vi "SEA_9811_RT_Driver_Tester.vi"() -> ()   [LabVIEW 2012]
uses:
  Typdefs/SEA9811_RT_conf_cluster.ctl
  <vilib>/userdefined/High Color/nirio_resource_hc.ctl
  FPGA/SEA-9811_ReceiverAndTransmitter/SubVIs/SEA-9811_ReceiverAndTransmitter_RCR.ctl
  FPGA/SEA-9811_ReceiverAndTransmitter/SubVIs/SEA-9811_ReceiverAndTransmitter_TCR.ctl
  FPGA/SEA-9811_ReceiverAndTransmitter/SubVIs/SEA-9811_ReceiverAndTransmitter_RSR.ctl
  Typdefs/ARINC word cluster.ctl
  Typdefs/ARINC word.ctl
  Typdefs/channel.ctl
  Typdefs/received word.ctl
  <vilib>/Platform/TimedLoop/XDataNode/timing_clust.ctl
  <vilib>/Platform/TimedLoop/XDataNode/nitl_modes.ctl
  <vilib>/Platform/TimedLoop/XDataNode/wakeup.ctl
  <vilib>/Platform/TimedLoop/XDataNode/XDataNode.xnode
  <vilib>/Platform/TimedLoop/XDataNode/XDNodeRunTimeDep.lvlib
panel:
  in  "Run FPGA?":bool
  in  "Period (ms)":i64=5
  out "Channels":T1[](array[typedef]) {"Received Words"."word" format="%.0o"; "Received Words"."timestamp" format="%#.10g"}
  in  "ARINC word in":T3 {"ARINC word" format="%032b"}
  out "error out":errorcluster
  in  "stop 2":bool
  out "Receiver Status Register (RSR)":T5={"RSR0: FIFO channel 0 empty"=TRUE, "RSR1: FIFO channel 1 empty"=TRUE, "RSR2: FIFO channel 2 empty"=TRUE, "RSR3: FIFO channel 3 empty"=TRUE, "RSR4: FIFO channel 4 empty"=TRUE, "RSR5: FIFO channel 5 empty"=TRUE, "RSR6: FIFO channel 6 empty"=TRUE, "RSR7: FIFO channel 7 empty"=TRUE, "RSR8: FIFO channel 0 full"=FALSE, "RSR9: FIFO channel 1 full"=FALSE, "RSR10: FIFO channel 2 full"=FALSE, "RSR11: FIFO channel 3 full"=FALSE, "RSR12: FIFO channel 4 full"=FALSE, "RSR13: FIFO channel 5 full"=FALSE, "RSR14: FIFO channel 6 full"=FALSE, "RSR15: FIFO channel 7 full"=FALSE}
  out "DMA Overflow":bool
  in  "stop":bool
  in  "SEA9811_conf_cluster":T6={"FPGA resource name"="RIO0", "Rx ch conf (0..7)"=[{"Rx Channel Number (0..7)"=0, "Rx Label Filter"={"Label 00"=0, "Label 01"=0, "Label 02"=0, "Label 03"=0, "Label 04"=0, "Label 05"=0, "Label 06"=0, "Label 07"=0, "Label 08"=0, "Label 09"=0, "Label 10"=0, "Label 11"=0, "Label 12"=0, "Label 13"=0, "Label 14"=0, "Label 15"=0}, "Receiver Control Register (RCR)"={"RCR0: Data rate = ARINC 429 High-Speed (0) or Low-Speed (1)"=FALSE, "RCR1: not used"=FALSE, "RCR2: Label recognition for this channel enabled (1) or disabled (0)"=FALSE, "RCR3: Receiver channel disabled (1) or enabled (0)"=FALSE, "RCR4: Odd parity check for this channel enabled (1) or disabled (0"=FALSE, "RCR5: Receiver normal operation (1) or loopback mode (0)"=TRUE, "RCR6: Receiver Decoder disabled (0) or enabled (1) \n-> ARINC bits 10 and 9 must match RCR7 and RCR8"=FALSE, "RCR7: If receiver decoder is enabled (RCR6=1), \nthe ARINC bit 10 must match this bit"=FALSE, "RCR8: If receiver decoder is enabled (RCR6=1), \nthe ARINC bit 9 must match this bit"=FALSE, "RCR9: Label bit order for this channel non-reversed (1) \nor reversed (0)"=FALSE, "RCR10: not used"=FALSE, "RCR11: not used"=FALSE, "RCR12: not used"=FALSE, "RCR13: not used"=FALSE, "RCR14: not used"=FALSE, "RCR15: not used"=FALSE}}, {"Rx Channel Number (0..7)"=3, "Rx Label Filter"={"Label 00"=23, "Label 01"=34, "Label 02"=0, "Label 03"=0, "Label 04"=0, "Label 05"=0, "Label 06"=0, "Label 07"=0, "Label 08"=0, "Label 09"=0, "Label 10"=0, "Label 11"=0, "Label 12"=0, "Label 13"=0, "Label 14"=0, "Label 15"=0}, "Receiver Control Register (RCR)"={"RCR0: Data rate = ARINC 429 High-Speed (0) or Low-Speed (1)"=FALSE, "RCR1: not used"=FALSE, "RCR2: Label recognition for this channel enabled (1) or disabled (0)"=FALSE, "RCR3: Receiver channel disabled (1) or enabled (0)"=FALSE, "RCR4: Odd parity check for this channel enabled (1) or disabled (0"=FALSE, "RCR5: Receiver normal operation (1) or loopback mode (0)"=TRUE, "RCR6: Receiver Decoder disabled (0) or enabled (1) \n-> ARINC bits 10 and 9 must match RCR7 and RCR8"=FALSE, "RCR7: If receiver decoder is enabled (RCR6=1), \nthe ARINC bit 10 must match this bit"=FALSE, "RCR8: If receiver decoder is enabled (RCR6=1), \nthe ARINC bit 9 must match this bit"=FALSE, "RCR9: Label bit order for this channel non-reversed (1) \nor reversed (0)"=FALSE, "RCR10: not used"=FALSE, "RCR11: not used"=FALSE, "RCR12: not used"=FALSE, "RCR13: not used"=FALSE, "RCR14: not used"=FALSE, "RCR15: not used"=FALSE}}, {"Rx Channel Number (0..7)"=5, "Rx Label Filter"={"Label 00"=2, "Label 01"=3, "Label 02"=0, "Label 03"=0, "Label 04"=0, "Label 05"=0, "Label 06"=0, "Label 07"=0, "Label 08"=0, "Label 09"=0, "Label 10"=0, "Label 11"=0, "Label 12"=0, "Label 13"=0, "Label 14"=0, "Label 15"=0}, "Receiver Control Register (RCR)"={"RCR0: Data rate = ARINC 429 High-Speed (0) or Low-Speed (1)"=FALSE, "RCR1: not used"=FALSE, "RCR2: Label recognition for this channel enabled (1) or disabled (0)"=FALSE, "RCR3: Receiver channel disabled (1) or enabled (0)"=FALSE, "RCR4: Odd parity check for this channel enabled (1) or disabled (0"=FALSE, "RCR5: Receiver normal operation (1) or loopback mode (0)"=TRUE, "RCR6: Receiver Decoder disabled (0) or enabled (1) \n-> ARINC bits 10 and 9 must match RCR7 and RCR8"=FALSE, "RCR7: If receiver decoder is enabled (RCR6=1), \nthe ARINC bit 10 must match this bit"=FALSE, "RCR8: If receiver decoder is enabled (RCR6=1), \nthe ARINC bit 9 must match this bit"=FALSE, "RCR9: Label bit order for this channel non-reversed (1) \nor reversed (0)"=FALSE, "RCR10: not used"=FALSE, "RCR11: not used"=FALSE, "RCR12: not used"=FALSE, "RCR13: not used"=FALSE, "RCR14: not used"=FALSE, "RCR15: not used"=FALSE}}], "Transmitter Control Register (TCR)"={"TCR0: not used"=FALSE, "TCR1: not used"=FALSE, "TCR2: not used"=FALSE, "TCR3: Transmitter Parity Bit Enable: 32nd bit is parity (1) or data (0)"=FALSE, "TCR4: not used"=FALSE, "TCR5: not used"=FALSE, "TCR6: not used"=FALSE, "TCR7: not used"=FALSE, "TCR8: not used"=FALSE, "TCR9: Transmitter Parity Select: odd parity (0) or even parity (1)"=FALSE, "TCR10: Transmitter Data Rate: ARINC 429 high-speed (0) or low-speed (1)"=FALSE, "TCR11: ARINC Label Bit Order: label bit order reversed (0) or not reversed (1)"=FALSE, "TCR12: Disable Line Driver: normal operation (0) or transmitter disabled (1)"=FALSE, "TCR13: Tansmit whenever data is available in FIFO (1) or only start by instruction \"Enable Transmission\" (0)"=TRUE, "TCR14: not used"=FALSE, "TCR15: not used"=FALSE}, "Bitfile Path"=path "c:/SEA-9811_ReceiverAndTransmitter_FPGA_IO_simulated.vi.lvbitx"}
  # "Run FPGA VI directly for interactive execution! Otherwise set Run FPGA? to TRUE"
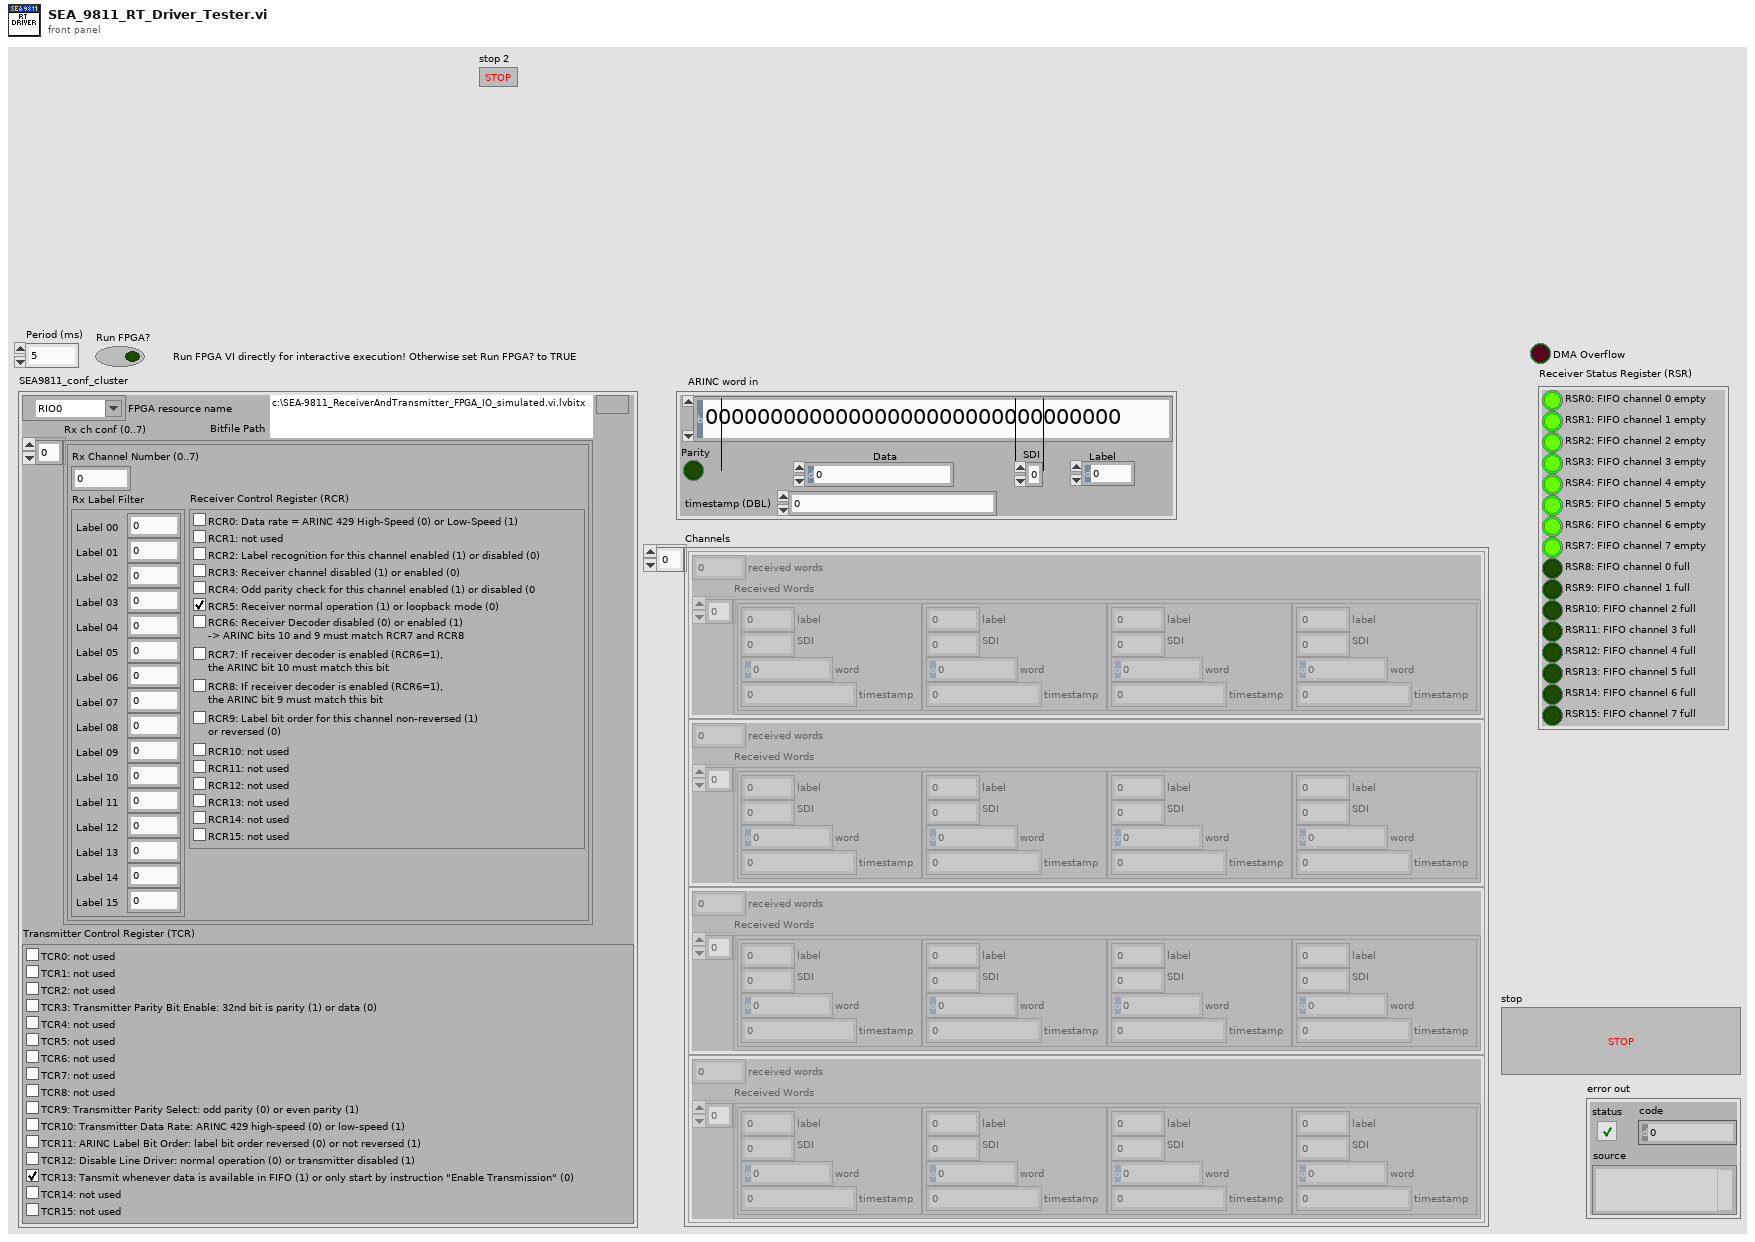
[diagram p1: front panel]
types:
  T1 = typedef "channel.ctl" = cluster{"received words":u32, "Received Words":T2[]}
  T2 = typedef "received word.ctl" = cluster{"label":u8, "SDI":u8, "word":u32, "timestamp":dbl}
  T3 = typedef "ARINC word cluster.ctl" = cluster{"ARINC word":T4, "Label":u8, "SDI":u8, "Data":u32, "Parity":bool, "timestamp (DBL)":dbl}
  T4 = typedef "ARINC word.ctl" = u32
  T5 = typedef "SEA-9811_ReceiverAndTransmitter_RSR.ctl" = cluster{"RSR0: FIFO channel 0 empty":bool, "RSR1: FIFO channel 1 empty":bool, "RSR2: FIFO channel 2 empty":bool, "RSR3: FIFO channel 3 empty":bool, "RSR4: FIFO channel 4 empty":bool, "RSR5: FIFO channel 5 empty":bool, "RSR6: FIFO channel 6 empty":bool, "RSR7: FIFO channel 7 empty":bool, "RSR8: FIFO channel 0 full":bool, "RSR9: FIFO channel 1 full":bool, "RSR10: FIFO channel 2 full":bool, "RSR11: FIFO channel 3 full":bool, "RSR12: FIFO channel 4 full":bool, "RSR13: FIFO channel 5 full":bool, "RSR14: FIFO channel 6 full":bool, "RSR15: FIFO channel 7 full":bool}
  T6 = typedef "SEA9811_RT_conf_cluster.ctl" = cluster{"FPGA resource name":T7, "Rx ch conf (0..7)":cluster{"Rx Channel Number (0..7)":u8, "Rx Label Filter":cluster{"Label 00":u8, "Label 01":u8, "Label 02":u8, "Label 03":u8, "Label 04":u8, "Label 05":u8, "Label 06":u8, "Label 07":u8, "Label 08":u8, "Label 09":u8, "Label 10":u8, "Label 11":u8, "Label 12":u8, "Label 13":u8, "Label 14":u8, "Label 15":u8}, "Receiver Control Register (RCR)":T8}[], "Transmitter Control Register (TCR)":T9, "Bitfile Path":path}
  T7 = typedef "nirio_resource_hc.ctl" = tag
  T8 = typedef "SEA-9811_ReceiverAndTransmitter_RCR.ctl" = cluster{"RCR0: Data rate = ARINC 429 High-Speed (0) or Low-Speed (1)":bool, "RCR1: not used":bool, "RCR2: Label recognition for this channel enabled (1) or disabled (0)":bool, "RCR3: Receiver channel disabled (1) or enabled (0)":bool, "RCR4: Odd parity check for this channel enabled (1) or disabled (0":bool, "RCR5: Receiver normal operation (1) or loopback mode (0)":bool, "RCR6: Receiver Decoder disabled (0) or enabled (1) \n-> ARINC bits 10 and 9 must match RCR7 and RCR8":bool, "RCR7: If receiver decoder is enabled (RCR6=1), \nthe ARINC bit 10 must match this bit":bool, "RCR8: If receiver decoder is enabled (RCR6=1), \nthe ARINC bit 9 must match this bit":bool, "RCR9: Label bit order for this channel non-reversed (1) \nor reversed (0)":bool, "RCR10: not used":bool, "RCR11: not used":bool, "RCR12: not used":bool, "RCR13: not used":bool, "RCR14: not used":bool, "RCR15: not used":bool}
  T9 = typedef "SEA-9811_ReceiverAndTransmitter_TCR.ctl" = cluster{"TCR0: not used":bool, "TCR1: not used":bool, "TCR2: not used":bool, "TCR3: Transmitter Parity Bit Enable: 32nd bit is parity (1) or data (0)":bool, "TCR4: not used":bool, "TCR5: not used":bool, "TCR6: not used":bool, "TCR7: not used":bool, "TCR8: not used":bool, "TCR9: Transmitter Parity Select: odd parity (0) or even parity (1)":bool, "TCR10: Transmitter Data Rate: ARINC 429 high-speed (0) or low-speed (1)":bool, "TCR11: ARINC Label Bit Order: label bit order reversed (0) or not reversed (1)":bool, "TCR12: Disable Line Driver: normal operation (0) or transmitter disabled (1)":bool, "TCR13: Tansmit whenever data is available in FIFO (1) or only start by instruction \"Enable Transmission\" (0)":bool, "TCR14: not used":bool, "TCR15: not used":bool}
  T10 = typedef "SEA9811_RT_data_cluster.ctl" = cluster{"FPGA VI Reference":T11, "Channels":T1[], "FPGA FP":T12, "Tx":cluster{"Tx Refs (Data,Trig)":T13[], "Values":dbl[]}}
  T11 = typedef "FPGA ref.ctl" = refnum<k20>
  T12 = typedef "SEA9811_FPGA_FP_Addresses.ctl" = cluster{"FPGA Interface Base on":refnum<class "FPGA Interface Base.lvclass">, "FPGA Session":u32, "RT time (ns)":u32, "DMA Overflow":u32, "Elements in FIFO":u32, "Rx Status":u32, "Rx Data (FIFO)":u32, "Tx Data":u32, "Transmit Data":u32}
  T13 = typedef "Custom Device API.lvlib/Block Data Reference.ctl" = cluster{"Data Reference":T14, "Offset":i32, "Length":i32}
  T14 = typedef "Custom Device API.lvlib/Data Reference.ctl" = i32
  T15 = typedef "XDNodeRunTimeDep.lvlib/timing_clust.ctl" = cluster{"Expected End [f-1]":u64, "Actual End [f-1]":u64, "Finished Late? [f-1]":bool, "Expected End [i-1]":u64, "Actual End [i-1]":u64, "Finished Late? [i-1]":bool, "Expected Start [i]":u64, "Actual Start [i]":u64, "Expected Start [f]":u64, "Actual Start [f]":u64, "Source Name":string, "Structure Name":string, "Period":i64, "Deadline":i64, "Offset":i64, "Start":i64, "Priority":i32, "Timeout":i32, "Mode":T16, "Wakeup Reason":T17, "Error":errorcluster, "Source Type":string, "Secondary Source Type":string, "Global End Time":u64, "Global Start Time":u64, "Frame Duration":u64, "Iteration Duration":u64, "Assigned CPU":i32, "I/O Scan Engine Mode":u32}
  T16 = typedef "XDNodeRunTimeDep.lvlib/nitl_modes.ctl" = enum32{"No Change", "Process missed periods, maintain original phase", "Discard missed periods, maintain original phase", "Process missed periods, ignore original phase", "Discard missed periods, ignore original phase"}
  T17 = typedef "XDNodeRunTimeDep.lvlib/wakeup.ctl" = enum32{"Normal", "Aborted", "Asynchronous wakeup", "Timing source error", "Timed loop error", "Timeout"}
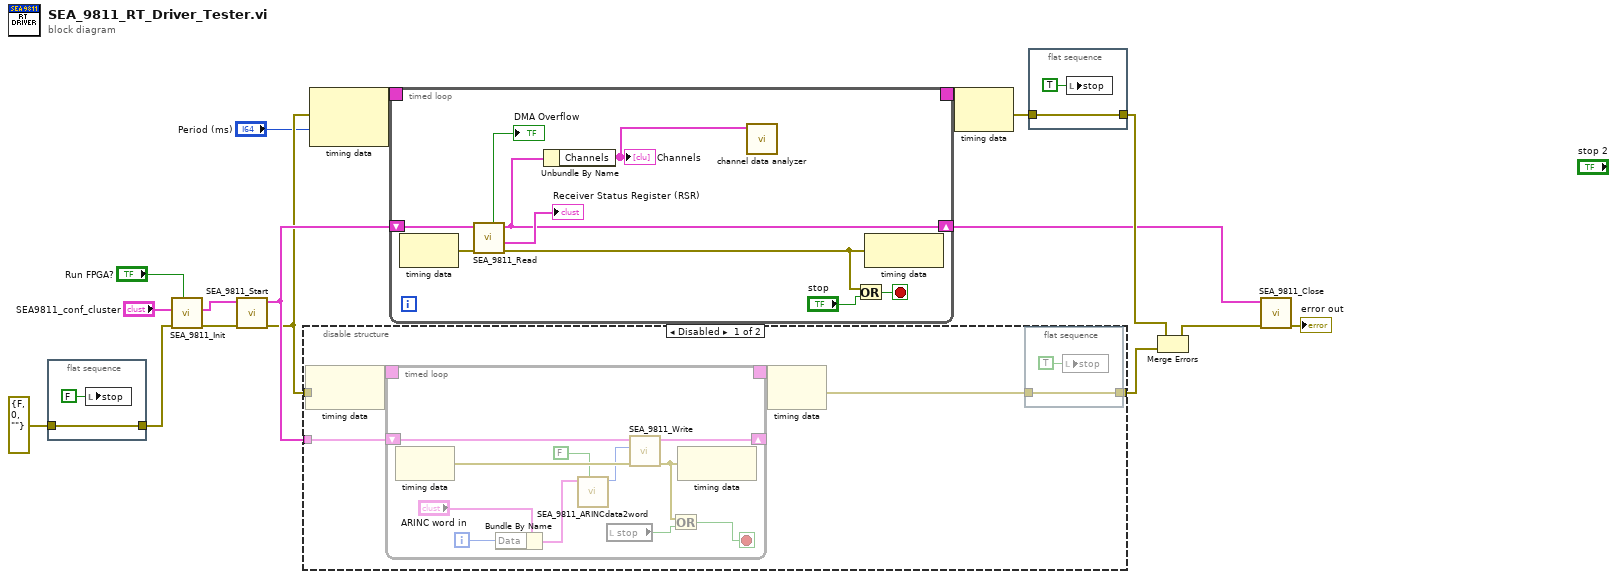
[diagram p0: block diagram]
diagram:
  n1 = flat-sequence {
    tunnel: errorcluster {"status"=FALSE, "code"=0, "source"=""} ("error in") -> [w18]
    tunnel: [w18] -> w11
    frame #0 {
      n2 = local write "stop"(FALSE ("stop")) -> ()
    }
  }
  n3 = call "SEA_9811_Init.vi"("Run?"="Run FPGA?", "error in"=w11, "SEA9811_conf_cluster"="SEA9811_conf_cluster") -> ("error out"=w17:errorcluster, "SEA9811_RT_data out"=w3:T10)  [unwired: 6 in, 1 out]
  n4 = call "SEA_9811_Start.vi"("error in (no error)"=w17, "SEA9811_RT_data in"=w3) -> ("error out"=w13:errorcluster, "SEA9811_RT_data out"=w16:T10)  [unwired: 8 in]
  n5 = disable-structure shown="Disabled" {
    disable-tunnel: w16 -> [w23 _]
    disable-tunnel: w13 -> [w22 w49]
    disable-tunnel: [w20 w49] -> w8
    frame Disabled {
      n6 = node-c288(w22) -> (w25:T15)
      n7 = timed-loop {
        timing: w25 -> [_]
        timing-out: [_] -> w24
        shift-right: [w31] -> _
        shift-left: w23 -> [w36]
        i -> [w29]
        stop <- w32 stop-if-true
        n8 = node-c288() -> (w35:errorcluster)  [unwired: 1 in]
        n9 = Bundle By Name(cluster="ARINC word in", "Data"=w29) -> (w27:T3)
        n10 = call "SEA_9811_ARINCdata2word.vi"("Reverse label bits"=FALSE, "ARINC word in"=w27) -> ("ARINC word out"=w30:T4)  [unwired: 8 in, 1 out]
        n11 = local read "stop"() -> (w34:bool)
        n12 = call "SEA_9811_Write.vi"("error in (no error)"=w35, "Tx Data"=w30, "SEA9811_RT_data in"=w36) -> ("error out"=w33:errorcluster, "SEA9811_RT_data out"=w31:T10)  [unwired: 7 in]
        n13 = Or(x=w33, y=w34) -> (x .or. y?=w32:bool)
        n14 = node-c288(w33) -> ()  [unwired: 1 out]
      }
      n15 = node-c288(w24) -> (w21:errorcluster)
      n16 = flat-sequence {
        tunnel: w21 -> [w47]
        tunnel: [w47] -> w20
        frame #0 {
          n17 = local write "stop"(TRUE ("stop")) -> ()
        }
      }
    }
    frame Enabled {
      # "write not implemented in dynamic bitfile version"
    }
  }
  n18 = node-c288(w13, "Period (ms)") -> (w15:T15)
  n19 = timed-loop {
    timing: w15 -> [_]
    timing-out: [_] -> w14
    shift-right: [w51] -> w6
    shift-left: w16 -> [w58]
    stop <- w55 stop-if-true
    n20 = node-c288() -> (w57:errorcluster)  [unwired: 1 in]
    n21 = call "SEA_9811_Read.vi"("error in (no error)"=w57, "SEA9811_RT_data in"=w58) -> ("error out"=w52:errorcluster, "Receiver Status Register (RSR)"=→"Receiver Status Register (RSR)":T5, "SEA9811_RT_data out"=w51:T10, "DMA Overflow"=→"DMA Overflow":bool)  [unwired: 6 in]
    n22 = Unbundle By Name(w51) -> ("Channels"=w50:T1[])
    "Channels" <- w50
    n23 = call "channel data analyzer.vi"("Channels"=w50) -> ()  [unwired: 11 in]
    n24 = Or(x=w52, y="stop") -> (x .or. y?=w55:bool)
    n25 = node-c288(w52) -> ()  [unwired: 1 out]
  }
  n26 = node-c288(w14) -> (w10:errorcluster)
  n27 = flat-sequence {
    tunnel: w10 -> [w64]
    tunnel: [w64] -> w9
    frame #0 {
      n28 = local write "stop"(TRUE ("stop")) -> ()
    }
  }
  n29 = Merge Errors(w9, w8) -> (w7:errorcluster)
  n30 = call "SEA_9811_Close.vi"("error in (no error)"=w7, "SEA9811_RT_data in"=w6) -> ("error out"=→"error out":errorcluster)  [unwired: 9 in]
